vi "Monty_Hall_Yiran.vi"() -> ()   [LabVIEW 2025]
panel:
  out "Possibility to win for 100 rounds":dbl
  out "?":dbl
  out "Possibility to win for Stay Strategy":dbl
  in  "Number of doors(up to 10)":dbl
  # "Possibility to win for Switch Strategy"
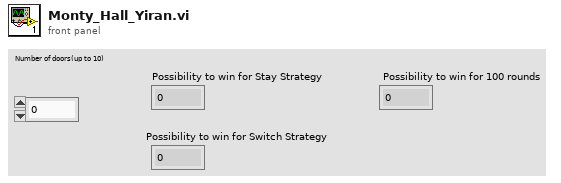
[diagram p1: front panel]
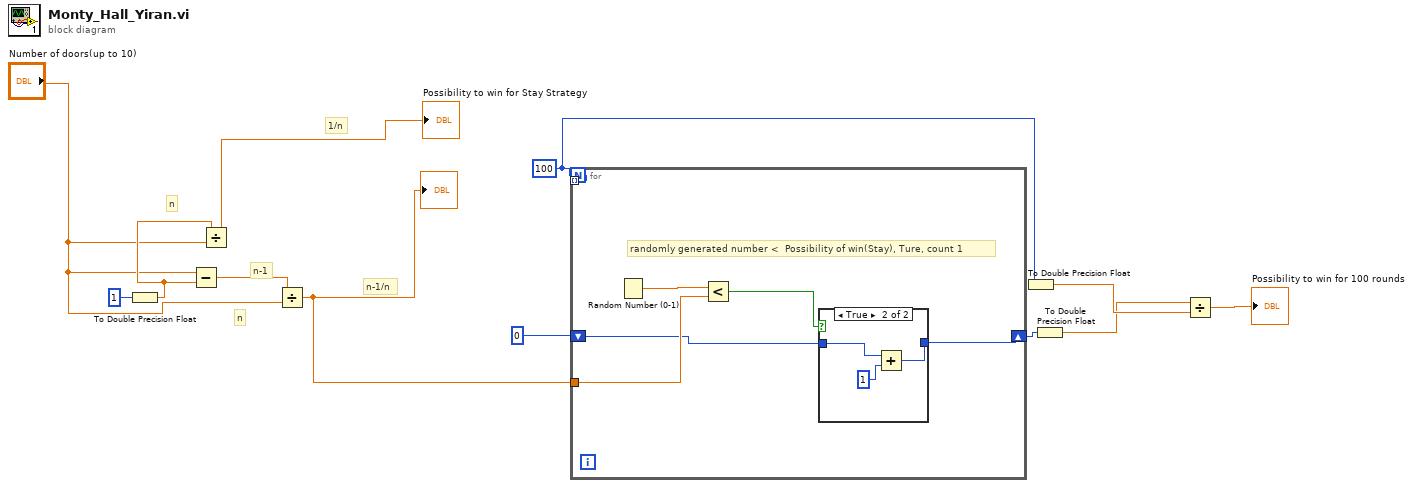
[diagram p0: block diagram]
diagram:
  w6 = 100
  # "1/n"
  # "n-1/n"
  # "n"
  # "n-1"
  # "n"
  n1 = To Double Precision Float(number=1) -> (double precision float=w10:dbl)
  n2 = Subtract(x="Number of doors(up to 10)", y=w10) -> (x-y=w11:dbl)
  n3 = Divide(x=w10, y="Number of doors(up to 10)") -> (x/y=→"Possibility to win for Stay Strategy":dbl)
  n4 = Divide(x=w11, y="Number of doors(up to 10)") -> (x/y=w8:dbl)
  "?" <- w8
  n5 = for {
    N: w6 -> [w18]
    tunnel: [w18] -> _ mode=indexing
    shift-right: [w14] -> w5
    shift-left: 0 -> [w15]
    tunnel: w8 -> [w16]
    # "randomly generated number <  Possibility of win(Stay), Ture, count 1"
    n6 = Random Number (0-1)() -> (number: 0 to 1=w17:dbl)
    n7 = Less?(x=w17, y=w16) -> (x < y?=w13:bool)
    n8 = case shown="True" w13 {
      tunnel: [w19 w20] -> w14
      tunnel: w15 -> [w19 w22]
      frame False {
      }
      frame True {
        n9 = Add(x=w22, y=1) -> (x+y=w20:i32)
      }
    }
  }
  n10 = To Double Precision Float(number=w6) -> (double precision float=w4:dbl)
  n11 = To Double Precision Float(number=w5) -> (double precision float=w3:dbl)
  n12 = Divide(x=w3, y=w4) -> (x/y=→"Possibility to win for 100 rounds":dbl)
